vi "Step Mode - Set Configurations.vi"   [LabVIEW 2014, in "Associated Power Technologies 8500 Series.lvlib"]
uses:
  <instrlib>/Associated Power Technologies 8500 Series/Associated Power Technologies 8500 Series.lvlib
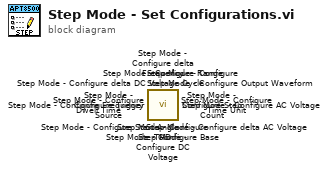
[diagram p0: block diagram]
diagram:
  n1 = call <instrlib>:"Step Mode - Configure THD.vi"() -> ()  [unwired: 10 in, 2 out]
  n2 = call <instrlib>:"Step Mode - Configure Cycle.vi"() -> ()  [unwired: 10 in, 2 out]
  n3 = call <instrlib>:"Step Mode - Configure Dwell Time.vi"() -> ()  [unwired: 10 in, 2 out]
  n4 = call <instrlib>:"Step Mode - Configure Time Unit.vi"() -> ()  [unwired: 10 in, 2 out]
  n5 = call <instrlib>:"Step Mode - Configure delta DC Voltage.vi"() -> ()  [unwired: 10 in, 2 out]
  n6 = call <instrlib>:"Step Mode - Configure delta Frequency.vi"() -> ()  [unwired: 10 in, 2 out]
  n7 = call <instrlib>:"Step Mode - Configure delta AC Voltage.vi"() -> ()  [unwired: 10 in, 2 out]
  n8 = call <instrlib>:"Step Mode - Configure DC Voltage.vi"() -> ()  [unwired: 10 in, 2 out]
  n9 = call <instrlib>:"Step Mode - Configure Frequency.vi"() -> ()  [unwired: 10 in, 2 out]
  n10 = call <instrlib>:"Step Mode - Configure AC Voltage.vi"() -> ()  [unwired: 10 in, 2 out]
  n11 = call <instrlib>:"Step Mode - Configure Start Angle.vi"() -> ()  [unwired: 10 in, 2 out]
  n12 = call <instrlib>:"Step Mode - Configure Output Waveform.vi"() -> ()  [unwired: 10 in, 2 out]
  n13 = call <instrlib>:"Step Mode - Configure Range.vi"() -> ()  [unwired: 10 in, 2 out]
  n14 = call <instrlib>:"Step Mode - Configure Base.vi"() -> ()  [unwired: 10 in, 2 out]
  n15 = call <instrlib>:"Step Mode - Configure Trigger Source.vi"() -> ()  [unwired: 10 in, 2 out]
  n16 = call <instrlib>:"Step Mode - Configure Step Count.vi"() -> ()  [unwired: 10 in, 2 out]
